vi "CRYProbe Window Close.vi"   [LabVIEW 2013]
uses:
  Global/CRYCurve Library Global.vi
panel:
  # "Close Probe Windows"
types:
  T1 = cluster{"Type Name":string, "Data Name":string, "Probe VIRef Number":i32, "Probe VIRef":refnum<vi>}[]
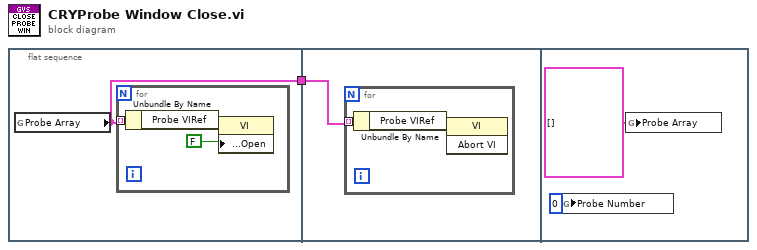
[diagram p0: block diagram]
diagram:
  n1 = flat-sequence {
    tunnel: [w2] -> w1
    tunnel: w1 -> [w6]
    frame #0 {
      n2 = global read "CRYCurve Library Global.vi" "Probe Array"() -> (w2:T1)
      n3 = for {
        tunnel: w2 -> [w4] mode=indexing
        n4 = Unbundle By Name(w4) -> ("Probe VIRef"=w3:refnum<vi>)
        n5 = property class="VI"(reference=w3, "Front Panel.Open"=FALSE ("Front Panel Window:Open")) -> ()  [unwired: 1 in, 2 out]
      }
    }
    frame #1 {
      n6 = for {
        tunnel: w6 -> [w8] mode=indexing
        n7 = Unbundle By Name(w8) -> ("Probe VIRef"=w7:refnum<vi>)
        n8 = invoke class="VI" method="Abort VI"(reference=w7) -> ()  [unwired: 2 in, 3 out]
      }
    }
    frame #2 {
      n9 = global write "CRYCurve Library Global.vi" "Probe Number"(0 ("Probe Number")) -> ()
      n10 = global write "CRYCurve Library Global.vi" "Probe Array"(T1 [] ("Probe Array")) -> ()
    }
  }
